vi "Pockels Cal-Generate required cal indexes.vi"(10 "Pockels calibration voltage steps sequence":dbl[](array[numeric])=[0.0, 0.05, 0.1, 0.15000000000000002, 0.2, 0.25, 0.3, 0.35, 0.39999999999999997, 0.44999999999999996, 0.49999999999999994, 0.5499999999999999, 0.6, 0.65, 0.7000000000000001, 0.7500000000000001, 0.8000000000000002, 0.8500000000000002, 0.9000000000000002, 0.9500000000000003, 1.0000000000000002], 11 "Parent FOR loop's index":i32=1) -> (2 "Required Cal indexes":i32[](array[numeric]))   [LabVIEW 2013]
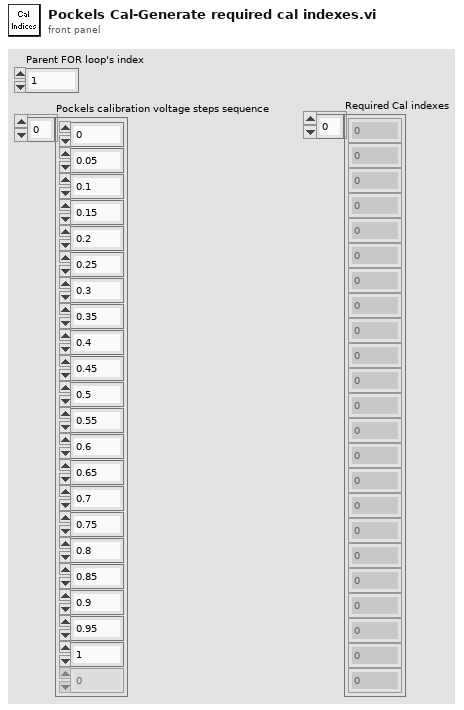
[diagram p1: front panel]
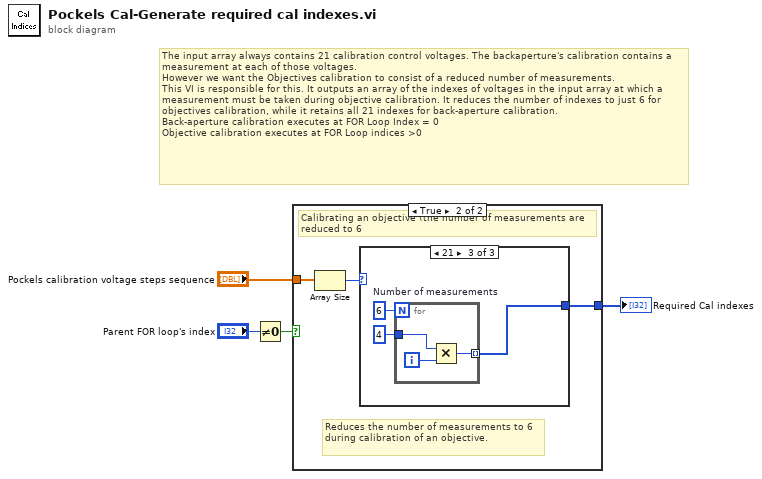
[diagram p0: block diagram]
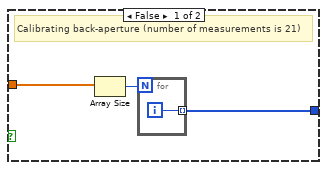
[diagram p2: hidden frame]
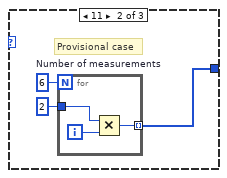
[diagram p4: hidden frame]
diagram:
  # "The input array always contains 21 calibration control voltages. The backaperture's calibration contains a measurement at each of those voltages.\nHowever we want the Objectives calibration to consist of a reduced number of measurements.\nThis VI is responsible for this. It outputs an array of the indexes of voltages in the input array at which a measurement must be taken during objective calibration. It reduces the number of indexes to just 6 for objectives calibration, while it retains all 21 indexes for back-aperture calibration.\nBack-aperture calibration executes at FOR Loop Index = 0\nObjective calibration executes at FOR Loop indices >0"
  n1 = Not Equal To 0?(x="Parent FOR loop's index") -> (x != 0?=w4:bool)
  n2 = case shown="True" w4 {
    tunnel: "Pockels calibration voltage steps sequence" -> [w6 w11]
    tunnel: [w7 w9] -> w3
    frame False {
      # "Calibrating back-aperture (number of measurements is 21)"
      n3 = Array Size(array=w6) -> (size(s)=w5:i32)
      n4 = for {
        N: w5 -> [_]
        tunnel: [w8] -> w7 mode=indexing
        i -> [w8]
      }
    }
    frame True {
      # "Reduces the number of measurements to 6 during calibration of an objective."
      # "Calibrating an objective (the number of measurements are reduced to 6"
      n5 = Array Size(array=w11) -> (size(s)=w10:i32)
      n6 = case shown="21" w10 {
        selector: w10 -> [w13 _ _]
        tunnel: [w12 w15 w21] -> w9
        frame Default {
          n7 = for {
            N: w13 -> [_]
            tunnel: [w14] -> w12 mode=indexing
            i -> [w14]
          }
        }
        frame 11 {
          w17 = 6  # Number of measurements
          # "Provisional case"
          n8 = for {
            N: w17 -> [_]
            tunnel: 2 -> [w19]
            tunnel: [w18] -> w15 mode=indexing
            i -> [w20]
            n9 = Multiply(x=w19, y=w20) -> (x*y=w18:i32)
          }
        }
        frame 21 {
          w23 = 6  # Number of measurements
          n10 = for {
            N: w23 -> [_]
            tunnel: 4 -> [w25]
            tunnel: [w24] -> w21 mode=indexing
            i -> [w26]
            n11 = Multiply(x=w25, y=w26) -> (x*y=w24:i32)
          }
        }
      }
    }
  }
  "Required Cal indexes" <- w3
